vi "Configure External Control.vi"(6 "Enable External Control State (False)":bool, 8 "error in (no error)":errorcluster, 9 "Enable Signal State (False)":bool, 10 "Signal (0)":u16(ring) items=["Input State", "Mode Control", "Setting", "Protection"], 11 "VISA resource name":refnum<visa-resource-name>) -> (0 "error out":errorcluster, 3 "VISA resource name out":refnum<visa-resource-name>)   [LabVIEW 2017, in "HH PLI Series.lvlib"]
doc: "Configures full external operation control over Analog I/O Port for specific input signals."
uses:
  HH PLI Series.lvlib
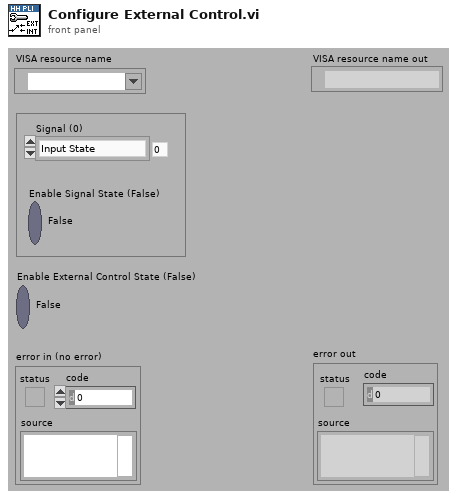
[diagram p1: front panel]
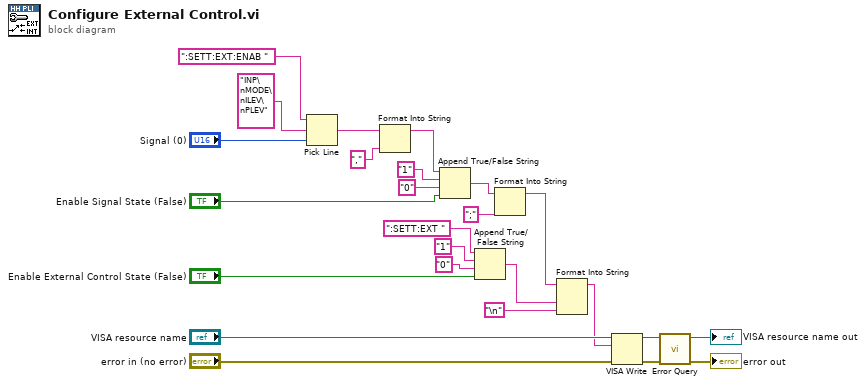
[diagram p0: block diagram]
diagram:
  n1 = Pick Line(string ("")=":SETT:EXT:ENAB " ("command"), multi-line string="INP\nMODE\nILEV\nPLEV" ("format string"), line index="Signal (0)") -> (output string=w8:string)
  n2 = Format Into String(initial string=w8, "," ("command")) -> (resulting string=w7:string)  [unwired: 2 in, 1 out]
  n3 = Append True/False String(1:"Enable Signal State (False)", 2:"0" ("false string"), 3:"1" ("true string"), 4:w7) -> (0:w5:string)
  n4 = Append True/False String(1:"Enable External Control State (False)", 2:"0" ("false string"), 3:"1" ("true string"), 4:":SETT:EXT " ("command")) -> (0:w2:string)
  n5 = Format Into String(initial string=w5, ";" ("string")) -> (resulting string=w3:string)  [unwired: 2 in, 1 out]
  n6 = Format Into String(initial string=w3, w2, "\n") -> (resulting string=w4:string)  [unwired: 2 in, 1 out]
  n7 = VISA Write(VISA resource name="VISA resource name", write buffer=w4, error in (no error)="error in (no error)") -> (VISA resource name out=w18:refnum<visa-resource-name>, error out=w19:errorcluster)  [unwired: 1 out]
  n8 = call "Error Query.vi"("error in (no error)"=w19, "VISA resource name"=w18) -> ("error out"=→"error out":errorcluster, "VISA resource name out"=→"VISA resource name out":refnum<visa-resource-name>)  [unwired: 6 in, 2 out]
